vi "GetSpeed.vi"(8 "error in (no error)":errorcluster, 11 "Bike in":refnum<class "Racer.lvclass">) -> (0 "error out":errorcluster, 2 "speed":dbl, 3 "Bike out":refnum<class "Racer.lvclass">)   [LabVIEW 2019, in "Racer.lvclass"]
doc: "Gets the speed.\n\nwww.sciware.com.au"
uses:
  Racer.lvclass
  Racer.lvclass/Racer.ctl
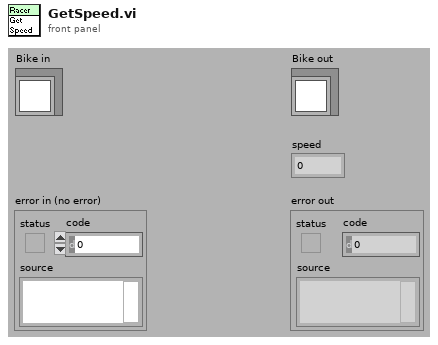
[diagram p1: front panel]
types:
  T1 = typedef "Racer.lvclass/DataRef.ctl" = refnum<data-value>
  T2 = typedef "Racer.lvclass/DataMembers.ctl" = cluster{"gear":i32}
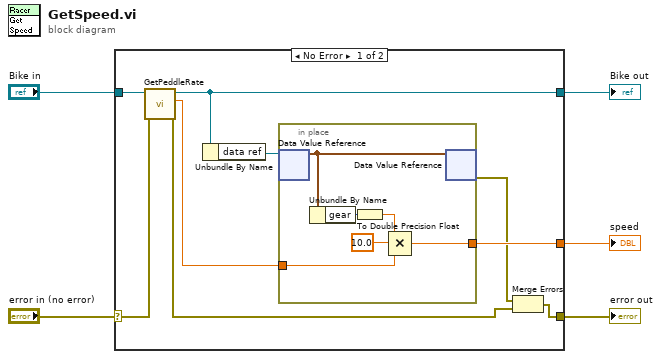
[diagram p0: block diagram]
diagram:
  n1 = case shown="No Error" "error in (no error)" {
    selector: "error in (no error)" -> [w10 w22]
    tunnel: [w8 w22] -> w4
    tunnel: [w11 w21] -> w2
    tunnel: "Bike in" -> [w12 w21]
    tunnel: [w13 _] -> w1
    frame No Error {
      n2 = call-dynamic "GetPeddleRate.vi"("error in (no error)"=w10, "Bike in"=w12) -> ("error out"=w9:errorcluster, "peddle rate"=w6:dbl, "Bike out"=w11:refnum<class "Racer.lvclass">)  [unwired: 7 in]
      n3 = Unbundle By Name(w11) -> ("data ref"=w14:T1)
      n4 = in-place {
        in-place-border: [w17] -> w13
        in-place-border: w6 -> [w15]
        n5 = in-place-dvr #1(w14) -> (w20:T2)  [unwired: 1 out]
        n6 = Unbundle By Name(w20) -> ("gear"=w19:i32)
        n7 = To Double Precision Float(number=w19) -> (double precision float=w16:dbl)
        n8 = Compound Arithmetic op=MULTIPLY(w16, 10.0 ("y"), w15) -> (w17:dbl)
        n9 = in-place-dvr #1(w20) -> (w7:errorcluster)  [unwired: 1 out]
      }
      n10 = Merge Errors(w7, w9) -> (w8:errorcluster)
    }
    frame Error {
    }
  }
  "error out" <- w4
  "Bike out" <- w2
  "speed" <- w1
